vi "Set_CleanSerialRegister.vi"(8 "error in":errorcluster, 10 "CleanSerialRegister":bool, 11 "camera handle in":u64) -> (0 "error out":errorcluster, 3 "camera handle out":u64)   [LabVIEW 2014, in "PICam.lvlib"]
doc: "Controls the number of rows in a clean cycle. The default value is equal with the Y pixel size of the CCD (for example, PIXIS400: 400)."
uses:
  PICam.lvlib
  Picam32.dll
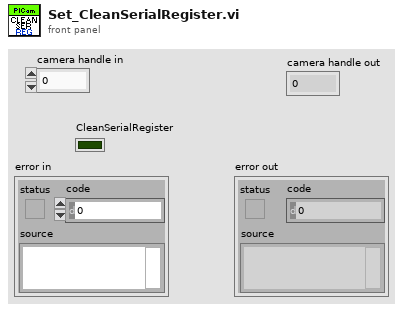
[diagram p1: front panel]
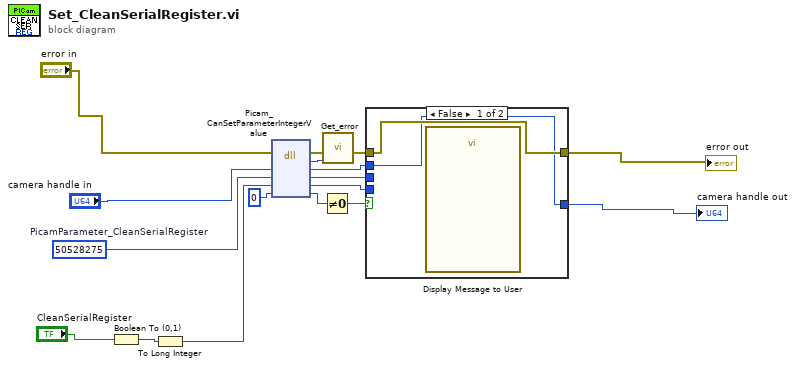
[diagram p0: block diagram]
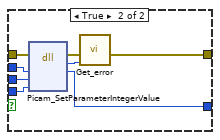
[diagram p2: hidden frame]
diagram:
  w9 = u32 50528275  # PicamParameter_CleanSerialRegister
  n1 = Boolean To (0,1)(Boolean="CleanSerialRegister") -> (0, 1=w2:i16)
  n2 = To Long Integer(number=w2) -> (32bit integer=w1:i32)
  n3 = dll-call lib="Picam32.dll" fn="Picam_CanSetParameterIntegerValue"(error in="error in", "camera"="camera handle in", "PicamParameter"=w9, "CleanSerialRegister"=w1, "bln"=0 ("CleanSerialRegister")) -> (error out=w16:errorcluster, "return type"=w17:i32, "camera"=w10:u64, "PicamParameter"=w8:u32, "CleanSerialRegister"=w13:i32, "bln"=w14:i32)  [unwired: 2 in, 1 out]
  n4 = Not Equal To 0?(x=w14) -> (x != 0?=w12:bool)
  n5 = call "Get_error.vi"("PICam_Error"=w17, "error in (no error)"=w16) -> ("error out"=w11:errorcluster)  [unwired: 9 in]
  n6 = case shown="False" w12 {
    tunnel: w13 -> [_ w25]
    tunnel: w11 -> [w19 w24]
    tunnel: w10 -> [w18 w23]
    tunnel: w8 -> [_ w22]
    tunnel: [w19 w21] -> w7
    tunnel: [w18 w20] -> w6
    frame False {
      n7 = call "Display Message to User"() -> ()  [unwired: 10 in, 2 out]
    }
    frame True {
      n8 = dll-call lib="Picam32.dll" fn="Picam_SetParameterIntegerValue"(error in=w24, "camera"=w23, "CleanSerialRegister"=w22, "TrackFrames"=w25) -> (error out=w27:errorcluster, "return type"=w26:i32, "camera"=w20:u64)  [unwired: 4 in, 1 out]
      n9 = call "Get_error.vi"("PICam_Error"=w26, "error in (no error)"=w27) -> ("error out"=w21:errorcluster)  [unwired: 9 in]
    }
  }
  "error out" <- w7
  "camera handle out" <- w6
